vi "RotateRect.vi"(8 "错误输入":errorcluster, 9 "90deg CW *":i16=1 caption="90度 CW *", 11 "rect":T1 caption="矩形") -> (0 "错误输出":errorcluster, 3 "rotated rect":T1 caption="旋转后的矩形")   [LabVIEW 2011, in "Rect Tools.lvlib"]
uses:
  Rect Tools.lvlib
panel:
  # "绕原点旋转"
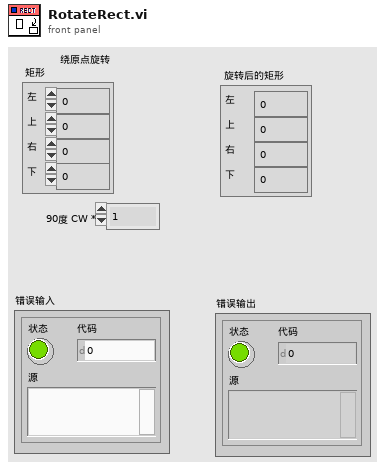
[diagram p1: front panel]
types:
  T1 = cluster{"left":i16, "top":i16, "right":i16, "bottom":i16}
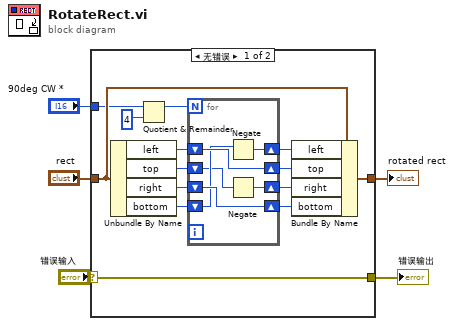
[diagram p0: block diagram]
diagram:
  n1 = case shown="无错误" "错误输入" {
    selector: "错误输入" -> [w9 w27]
    tunnel: [w9 w27] -> w4
    tunnel: "rect" -> [w8 w26]
    tunnel: [w7 w26] -> w2
    tunnel: "90deg CW *" -> [w6 _]
    frame No Error {
      n2 = Unbundle By Name(w8) -> ("left"=w17:i16, "top"=w16:i16, "right"=w15:i16, "bottom"=w14:i16)
      n3 = Quotient & Remainder(x=w6, y=i16 4) -> (x-y*floor(x/y)=w18:i16)  [unwired: 1 out]
      n4 = for {
        N: w18 -> [_]
        shift-right: [w22] -> w13
        shift-left: w17 -> [w25]
        shift-right: [w25] -> w12
        shift-left: w16 -> [w21]
        shift-right: [w20] -> w11
        shift-left: w15 -> [w24]
        shift-right: [w24] -> w10
        shift-left: w14 -> [w23]
        n5 = Negate(x=w23) -> (-x=w22:i16)
        n6 = Negate(x=w21) -> (-x=w20:i16)
      }
      n7 = Bundle By Name(cluster=w8, "left"=w13, "top"=w12, "right"=w11, "bottom"=w10) -> (w7:T1)
    }
    frame Error {
    }
  }
  "错误输出" <- w4
  "rotated rect" <- w2
